vi "Ctor.vi"(8 "error in (no error)":errorcluster, 11 "AppListPanel in":refnum<class "AppListPanel.lvclass">) -> (0 "error out":errorcluster, 3 "AppListPanel out":refnum<class "AppListPanel.lvclass">)   [LabVIEW 2020, in "PicoG-App.lvlib" / "AppListPanel.lvclass"]
uses:
  AppListPanel.lvclass
  Ref Data.ctl
  App Panel.ctl
  ViaApp/ViaApp.lvclass
  GWebAppArrayPanel/GWebAppArrayPanel.lvclass
  AppListPanel.lvclass/AppListPanel.ctl
  <vilib>/IlluminatedG/IG OOPanel/OOPanel/Panel/Panel.lvclass
  <vilib>/IlluminatedG/IG OOPanel/OOPanel/ArrayManager/ArrayManager.lvclass
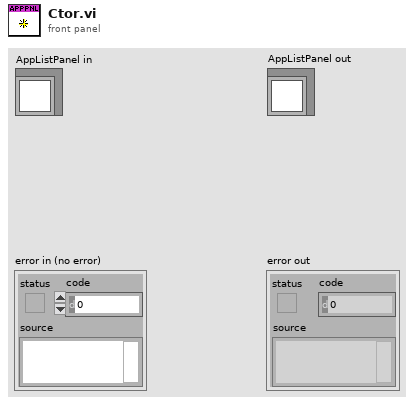
[diagram p1: front panel]
types:
  T1 = typedef "PicoG-App.lvlib/AppListPanel.lvclass/Ref Data.ctl" = cluster{"App Map":map{path, T2}}
  T2 = typedef "PicoG-App.lvlib/AppListPanel.lvclass/App Panel.ctl" = cluster{"App":refnum<class "ViaApp.lvclass">, "Panel":refnum<class "GWebAppArrayPanel.lvclass">}
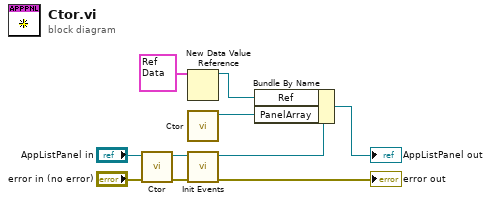
[diagram p0: block diagram]
diagram:
  n1 = call-parent <vilib>:"Ctor.vi"("error in (no error)"="error in (no error)", "Panel in"="AppListPanel in") -> ("error out"=w3:errorcluster, "Panel out"=w2:refnum<class "AppListPanel.lvclass">)  [unwired: 8 in]
  n2 = New Data Value Reference(data value=T1 {"App Map"={}} ("Ref Data")) -> (data value reference=w5:refnum<data-value>)  [unwired: 1 in, 1 out]
  n3 = call <vilib>:"Ctor.vi"() -> ("PanelArray"=w7:refnum<class "ArrayManager.lvclass">)  [unwired: 10 in, 1 out]
  n4 = call "Init Events.vi"("error in (no error)"=w3, "AppListPanel in"=w2) -> ("error out"=→"error out":errorcluster, "AppListPanel out"=w9:refnum<class "AppListPanel.lvclass">)  [unwired: 8 in]
  n5 = Bundle By Name(cluster=w9, "Ref"=w5, "PanelArray"=w7) -> (→"AppListPanel out":refnum<class "AppListPanel.lvclass">)
